vi "Register File Appender.vi"(8 "error in (no error)":errorcluster, 10 "FileAppenderConfig":T1={"common"={"id"="", "threshold"=enum."INFO", "filter"={"mode"=enum."Mirror", "levelMin"=enum."INFO", "levelMax"=enum."INFO", "tagPrefix"=""}, "queueBound"=-1, "dropPolicy"=enum."DropOldest", "useUTC"=FALSE}, "file"={"rootFolder"=path "", "maxFileSize"=-1, "maxFileCount"=-1, "baseName"="", "extension"="", "delimiter"="", "calendarFolderTree"=FALSE}}, 11 "Logger in":refnum<class "Logger.lvclass">) -> (0 "error out":errorcluster, 2 "id":string, 3 "Logger out":refnum<class "Logger.lvclass">)   [LabVIEW 2026, in "Tests.lvlib"]
doc: "Test Arrange step for file-mechanics tests. Registers a FileAppender with the running logger from a supplied FileAppenderConfig, blocking until it is live. The sink is on disk, so tests observe by reading files under the config's root folder after Shutdown flushes and closes them; this helper returns the id (from common.id) but no queue. Tests build the config from a default FileAppenderConfig constant, overriding file.rootFolder and common.id plus whichever mechanic they exercise (maxFileSize, maxFileCount, calendarFolderTree, filter)."
uses:
  Tests.lvlib
  src/Public/Logger.lvclass/Logger.lvclass
  src/TypeDefs/FileAppenderConfig.ctl
  src/TypeDefs/AppenderConfig.ctl
  src/TypeDefs/Severity.ctl
  src/TypeDefs/Filter.ctl
  src/TypeDefs/FilterMode.ctl
  src/TypeDefs/DropPolicy.ctl
  src/TypeDefs/FileConfig.ctl
  src/Core/Appenders/FileAppender.lvclass/FileAppender.lvclass
  src/Core/Layouts/CSVLayout.lvclass/CSVLayout.lvclass
  src/Lumberjack.lvlib
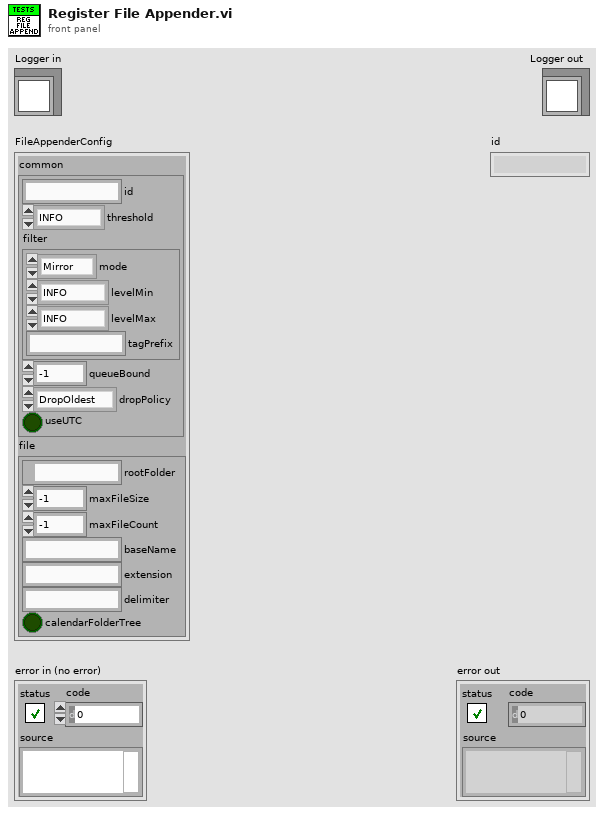
[diagram p1: front panel]
types:
  T1 = typedef "Lumberjack.lvlib/FileAppenderConfig.ctl" = cluster{"common":T2, "file":T7}
  T2 = typedef "Lumberjack.lvlib/AppenderConfig.ctl" = cluster{"id":string, "threshold":T3, "filter":T4, "queueBound":i32, "dropPolicy":T6, "useUTC":bool}
  T3 = typedef "Lumberjack.lvlib/Severity.ctl" = enum16{"OFF", "FATAL", "ERROR", "WARN", "INFO", "DEBUG", "TRACE", "ALL"}
  T4 = typedef "Lumberjack.lvlib/Filter.ctl" = cluster{"mode":T5, "levelMin":T3, "levelMax":T3, "tagPrefix":string}
  T5 = typedef "Lumberjack.lvlib/FilterMode.ctl" = enum16{"Mirror", "Routed"}
  T6 = typedef "Lumberjack.lvlib/DropPolicy.ctl" = enum16{"DropOldest", "DropNewest", "LevelAware"}
  T7 = typedef "Lumberjack.lvlib/FileConfig.ctl" = cluster{"rootFolder":path, "maxFileSize":i64, "maxFileCount":i32, "baseName":string, "extension":string, "delimiter":string, "calendarFolderTree":bool}
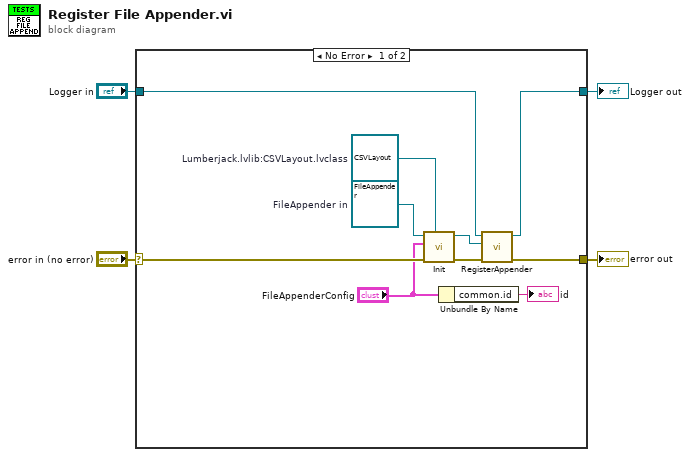
[diagram p0: block diagram]
diagram:
  n1 = case shown="No Error" "error in (no error)" {
    selector: "error in (no error)" -> [w14 w16]
    tunnel: [w11 w16] -> w3
    tunnel: [w12 w15] -> w1
    tunnel: "Logger in" -> [w13 w15]
    frame No Error {
      w5 = refnum<class "CSVLayout.lvclass"> refnum  # Lumberjack.lvlib:CSVLayout.lvclass
      w10 = refnum<class "FileAppender.lvclass"> refnum  # FileAppender in
      n2 = call "Init.vi"("Lumberjack.lvlib:Layout.lvclass"=w5, "error in (no error)"=w14, "FileAppenderConfig"="FileAppenderConfig", "FileAppender in"=w10) -> ("error out"=w8:errorcluster, "FileAppender out"=w9:refnum<class "FileAppender.lvclass">)  [unwired: 6 in]
      n3 = Unbundle By Name("FileAppenderConfig") -> ("common.id"=→"id":string)
      n4 = call "RegisterAppender.vi"("error in (no error)"=w8, "Lumberjack.lvlib:Appender.lvclass"=w9, "Logger in"=w13) -> ("error out"=w11:errorcluster, "Logger out"=w12:refnum<class "Logger.lvclass">)  [unwired: 7 in]
    }
    frame Error {
    }
  }
  "error out" <- w3
  "Logger out" <- w1
